vi "Init Editor Data.vi"(8 "error in":errorcluster) -> (0 "error out":errorcluster, 3 "TSC Button Editor":refnum<class "TSC Button Editor.lvclass">)   [LabVIEW 2021, in "TSC Button Editor.lvclass"]
uses:
  TSC Button Editor.lvclass
  TSC Button Editor.lvclass/TSC Button Editor.ctl
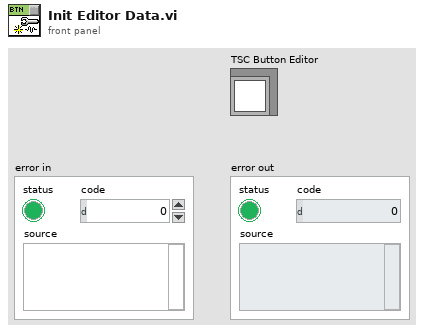
[diagram p1: front panel]
types:
  T1 = enum16{"open", "replace", "create", "open or create", "replace or create", "replace or create with confirmation"}
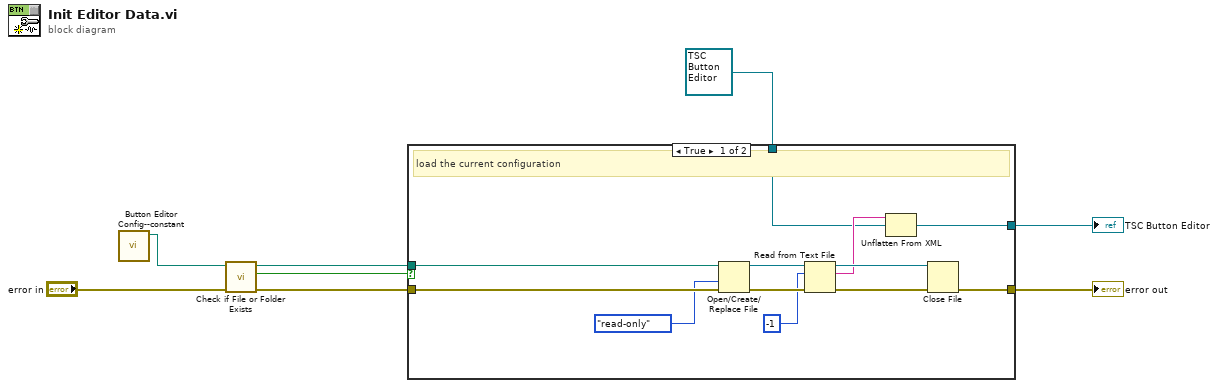
[diagram p0: block diagram]
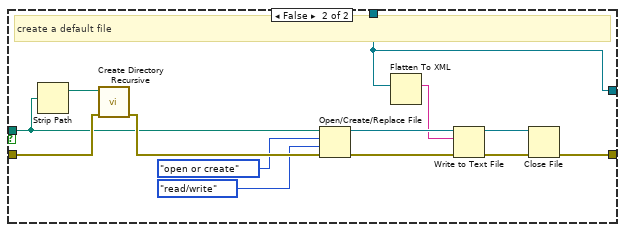
[diagram p2: hidden frame]
diagram:
  n1 = call "Button Editor Config--constant.vi"() -> ("Button Editor Config"=w5:path)  [unwired: 11 in]
  n2 = call <vilib>:"Check if File or Folder Exists.vi"("error in (no error)"="error in", "path"=w5) -> ("error out"=w7:errorcluster, "file or folder exists?"=w4:bool, "dup path"=w3:path)  [unwired: 7 in]
  n3 = case shown="True" w4 {
    tunnel: w7 -> [w20 w33]
    tunnel: w3 -> [w16 w21]
    tunnel: refnum<class "TSC Button Editor.lvclass"> refnum ("TSC Button Editor.lvclass") -> [w10 w23]
    tunnel: [w9 w23] -> w1
    tunnel: [w17 w30] -> w6
    frame True {
      # "load the current configuration"
      n4 = Open/Create/Replace File(file path (use dialog)=w16, error in=w20, access (0:read/write)=enum16{"read/write", "read-only", "write-only"}."read-only") -> (refnum out=w14:refnum<file>, error out=w19:errorcluster)  [unwired: 3 in, 1 out]
      n5 = Read from Text File(file (use dialog)=w14, count=-1, error in=w19) -> (refnum out=w12:refnum<file>, text=w11:string, error out=w18:errorcluster)  [unwired: 1 in, 1 out]
      n6 = Unflatten From XML(xml string=w11, type=w10) -> (value=w9:refnum<class "TSC Button Editor.lvclass">)  [unwired: 1 in, 1 out]
      n7 = Close File(refnum=w12, error in=w18) -> (error out=w17:errorcluster)  [unwired: 1 out]
    }
    frame False {
      # "create a default file"
      n8 = Strip Path(path=w21) -> (stripped path=w22:path)  [unwired: 1 out]
      n9 = call <vilib>:"Create Directory Recursive.vi"("error in (no error)"=w33, "directory"=w22) -> ("error out"=w29:errorcluster)  [unwired: 3 in, 2 out]
      n10 = Open/Create/Replace File(file path (use dialog)=w21, error in=w29, operation (0:open)=T1."open or create", access (0:read/write)=enum16{"read/write", "read-only", "write-only"}."read/write") -> (refnum out=w27:refnum<file>, error out=w32:errorcluster)  [unwired: 2 in, 1 out]
      n11 = Flatten To XML(6:w23) -> (2:w24:string)
      n12 = Write to Text File(file (use dialog)=w27, text=w24, error in=w32) -> (refnum out=w26:refnum<file>, error out=w31:errorcluster)  [unwired: 1 in, 1 out]
      n13 = Close File(refnum=w26, error in=w31) -> (error out=w30:errorcluster)  [unwired: 1 out]
    }
  }
  "error out" <- w6
  "TSC Button Editor" <- w1
